vi "Set IFD Entry.vi"(0 "Image Data in":u8[](array[numeric]), 1 "Offset in":i32, 2 "Tag":u16=30, 3 "Val / Offset":u32=106, 4 "Litt/BigEnd":bool) -> (5 "Image Data Out":u8[](array[numeric]), 6 "Directory Offset Out":i32, 7 "Replaced?":bool)   [LabVIEW 2013, in "Tiff reader.lvlib"]
doc: "Sets a tag entry in the Image File Directory in a tiff file byte stream."
uses:
  Tiff reader.lvlib
  IFD Entry.ctl
  FieldTypes.ctl
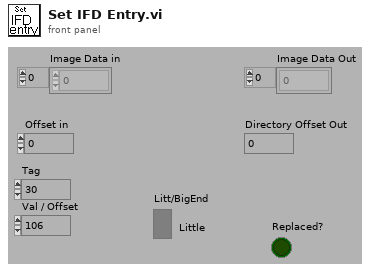
[diagram p1: front panel]
types:
  T1 = typedef "Tiff reader.lvlib/IFD Entry.ctl" = cluster{"Tag":u16, "Type":T2, "Count":u32, "Val/Offs":u32, "Is Pointer?":bool, "Byte stream index":i32}
  T2 = typedef "Tiff reader.lvlib/FieldTypes.ctl" = enum16{"NULL", "U8", "ASCII7", "U16", "U32", "RATIONAL", "SByte(I8)", "Undef(8Bit)", "I16", "I32", "SRat(4B:4B)", "SGL(4Byte)", "DBL(8Byte)"}
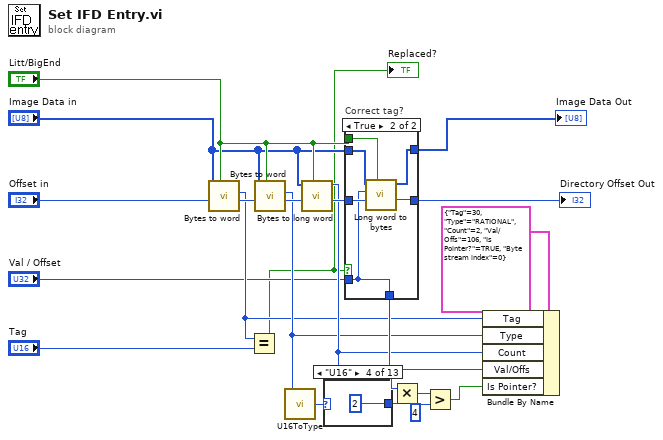
[diagram p0: block diagram]
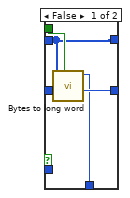
[diagram p2: hidden frame]
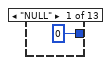
[diagram p3: hidden frame]
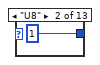
[diagram p4: hidden frame]
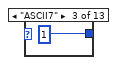
[diagram p5: hidden frame]
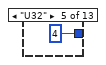
[diagram p6: hidden frame]
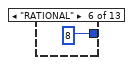
[diagram p7: hidden frame]
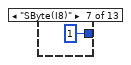
[diagram p8: hidden frame]
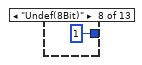
[diagram p9: hidden frame]
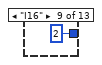
[diagram p10: hidden frame]
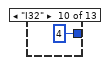
[diagram p11: hidden frame]
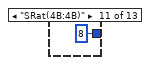
[diagram p12: hidden frame]
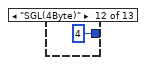
[diagram p13: hidden frame]
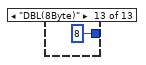
[diagram p14: hidden frame]
diagram:
  n1 = call "Bytes to word.vi"("Litt/BigEnd"="Litt/BigEnd", "Index"="Offset in", "Image Data in"="Image Data in") -> ("Index+2"=w19:i32, "Word"=w5:u16)  [unwired: 1 in, 4 out]
  n2 = Equal?(x=w5, y="Tag") -> (x = y?=w1:bool)
  "Replaced?" <- w1
  n3 = call "Bytes to word.vi"("Litt/BigEnd"="Litt/BigEnd", "Index"=w19, "Image Data in"="Image Data in") -> ("Index+2"=w18:i32, "Word"=w8:u16)  [unwired: 1 in, 4 out]
  n4 = call "U16ToType.vi"("U16 In"=w8) -> ("Type out"=w14:T2)  [unwired: 4 out]
  n5 = call "Bytes to long word.vi"("Litt/BigEnd"="Litt/BigEnd", "Index"=w18, "Image Data in"="Image Data in") -> ("Index+4"=w17:i32, "U32"=w12:u32)  [unwired: 5 out]
  n6 = case shown="\"U16\"" w14 {
    tunnel: [i64 0 i64 1 i64 1 i64 2 i64 4 i64 8 i64 1 i64 1 i64 2 i64 4 i64 8 i64 4 i64 8] -> w13
    frame "NULL" {
    }
    frame "U8" {
    }
    frame "ASCII7" {
    }
    frame "U16" {
    }
    frame "U32" {
    }
    frame "RATIONAL" {
    }
    frame "SByte(I8)" {
    }
    frame "Undef(8Bit)" {
    }
    frame "I16" {
    }
    frame "I32" {
    }
    frame "SRat(4B:4B)" {
    }
    frame "SGL(4Byte)" {
    }
    frame "DBL(8Byte)" {
    }
  }
  n7 = case "Correct tag?" shown="True" w1 {
    tunnel: w17 -> [w39 w45]
    tunnel: [w38 w41] -> w16
    tunnel: [w37 w40] -> w15
    tunnel: "Image Data in" -> [w35 w44]
    tunnel: "Litt/BigEnd" -> [w36 w43]
    tunnel: [w35 w42] -> w3
    tunnel: "Val / Offset" -> [_ w40]
    frame False {
      n8 = call "Bytes to long word.vi"("Litt/BigEnd"=w36, "Index"=w39, "Image Data in"=w35) -> ("Index+4"=w38:i32, "U32"=w37:u32)  [unwired: 5 out]
    }
    frame True {
      n9 = call "Long word to bytes.vi"("Litt/BigEnd"=w43, "Index"=w45, "U32"=w40, "Image Data in"=w44) -> ("Index+4"=w41:i32, "Image Data out"=w42:u8[])  [unwired: 4 out]
    }
  }
  "Directory Offset Out" <- w16
  "Image Data Out" <- w3
  n10 = Multiply(x=w12, y=w13) -> (x*y=w11:i64)
  n11 = Greater?(x=w11, y=i64 4) -> (0:w9:bool)
  n12 = Bundle By Name(cluster=T1 {"Tag"=30, "Type"=enum."RATIONAL", "Count"=2, "Val/Offs"=106, "Is Pointer?"=TRUE, "Byte stream index"=0} ("Cluster"), "Tag"=w5, "Type"=w8, "Count"=w12, "Val/Offs"=w15, "Is Pointer?"=w9) -> ()  [unwired: 1 out]
